vi "MoveXYZ.vi"(8 "error in (no error)":errorcluster, 9 "Destination coordinate":dbl[](array[numeric]), 10 "Notifiers":T1, 11 "Message Queues in":T14) -> (0 "error out":errorcluster)   [LabVIEW 2014]
uses:
  support/Message Queue/All Message Queues.ctl
  support/Message Queue/Message Cluster.ctl
  support/Notifiers/Notifiers.ctl
  support/Message Handler Loop Notifiers.ctl
  Parameter Analyzer/Parameter Analyzer Notifiers.ctl
  Switching Matrix/Switching Matrix Notifiers.ctl
  Stress Control/StressControl Notifiers.ctl
  Spectrometer/Spectrometer Notifiers.ctl
  Switches and Mirrors/SwitchesMirrors Notifiers.ctl
  Camera/Camera Notifiers.ctl
  XYZ Stage/XYZ Notifications.ctl
  Autofocus Notifiers.ctl
  Measurements/Optoelectronic Measurement/Optoelectronic Notifiers.ctl
  Measurements/Save Data/SaveData Notifiers.ctl
  Measurements/Instrument Sequence/Instrument Sequence Notifiers.ctl
  XYZ Stage/XYZ Config.ctl
  XYZ Stage/XYZ Connection Settings.ctl
  XYZ Stage/XYZ Stage Control.ctl
  XYZ Stage/XYZ Coordinate Control.ctl
  support/Message Queue/Message Queue.lvlib
panel:
  # "LICENSED MATERIALS – PROPERTY OF IBM\nCopyright IBM Corp. 2016, 2016\nALL RIGHTS RESERVED"
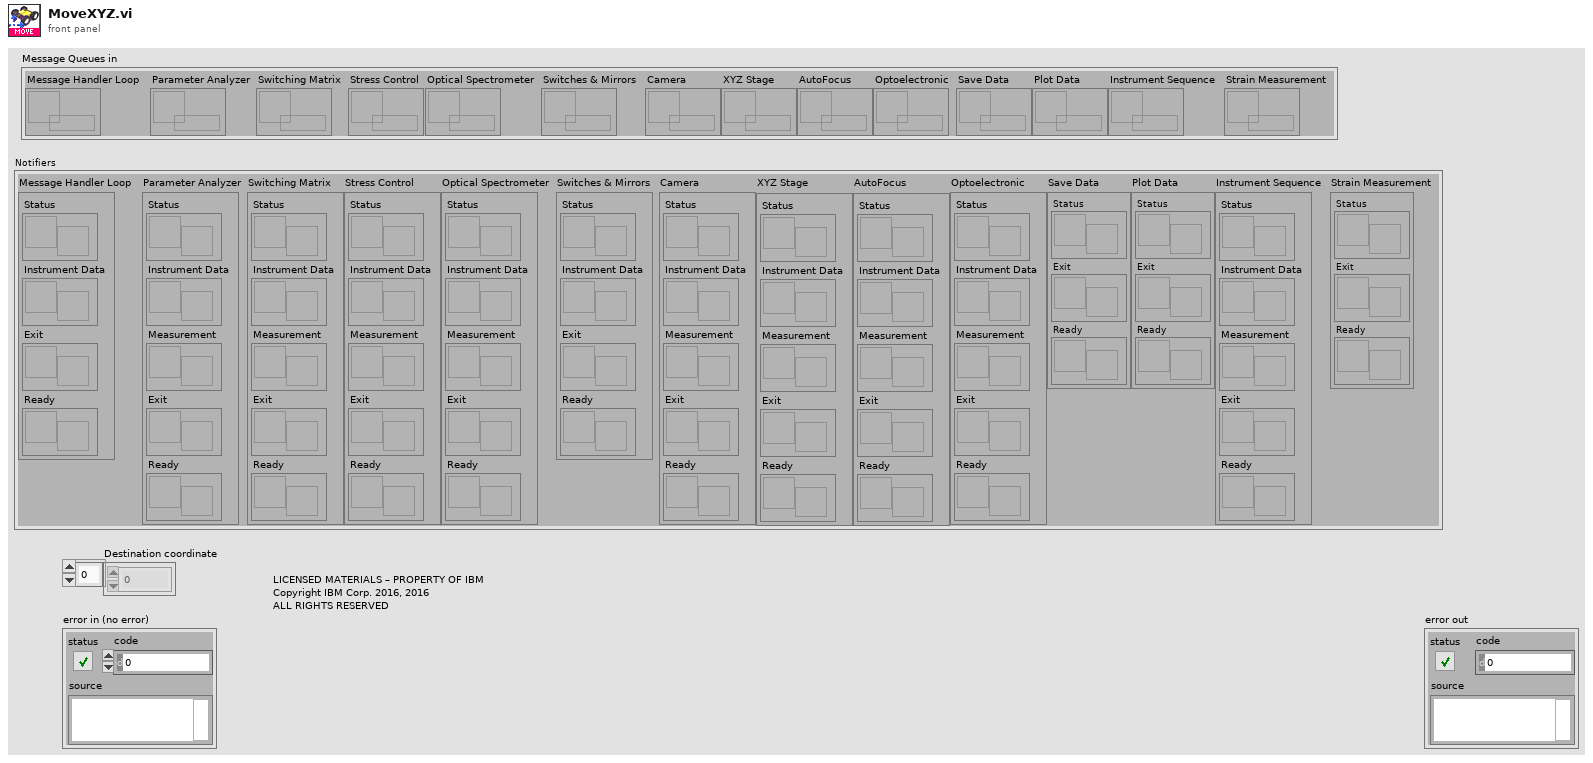
[diagram p1: front panel]
types:
  T1 = typedef "Notifiers.ctl" = cluster{"Message Handler Loop":T2, "Parameter Analyzer":T3, "Switching Matrix":T4, "Stress Control":T5, "Optical Spectrometer":T6, "Switches & Mirrors":T7, "Camera":T8, "XYZ Stage":T9, "AutoFocus":T10, "Optoelectronic":T11, "Save Data":T12, "Plot Data":T12, "Instrument Sequence":T13, "Strain Measurement":cluster{"Status":refnum<notifier>, "Exit":refnum<notifier>, "Ready":refnum<notifier>}}
  T2 = typedef "Message Handler Loop Notifiers.ctl" = cluster{"Status":refnum<notifier>, "Instrument Data":refnum<notifier>, "Exit":refnum<notifier>, "Ready":refnum<notifier>}
  T3 = typedef "Parameter Analyzer Notifiers.ctl" = cluster{"Status":refnum<notifier>, "Instrument Data":refnum<notifier>, "Measurement":refnum<notifier>, "Exit":refnum<notifier>, "Ready":refnum<notifier>}
  T4 = typedef "Switching Matrix Notifiers.ctl" = cluster{"Status":refnum<notifier>, "Instrument Data":refnum<notifier>, "Measurement":refnum<notifier>, "Exit":refnum<notifier>, "Ready":refnum<notifier>}
  T5 = typedef "StressControl Notifiers.ctl" = cluster{"Status":refnum<notifier>, "Instrument Data":refnum<notifier>, "Measurement":refnum<notifier>, "Exit":refnum<notifier>, "Ready":refnum<notifier>}
  T6 = typedef "Spectrometer Notifiers.ctl" = cluster{"Status":refnum<notifier>, "Instrument Data":refnum<notifier>, "Measurement":refnum<notifier>, "Exit":refnum<notifier>, "Ready":refnum<notifier>}
  T7 = typedef "SwitchesMirrors Notifiers.ctl" = cluster{"Status":refnum<notifier>, "Instrument Data":refnum<notifier>, "Exit":refnum<notifier>, "Ready":refnum<notifier>}
  T8 = typedef "Camera Notifiers.ctl" = cluster{"Status":refnum<notifier>, "Instrument Data":refnum<notifier>, "Measurement":refnum<notifier>, "Exit":refnum<notifier>, "Ready":refnum<notifier>}
  T9 = typedef "XYZ Notifications.ctl" = cluster{"Status":refnum<notifier>, "Instrument Data":refnum<notifier>, "Measurement":refnum<notifier>, "Exit":refnum<notifier>, "Ready":refnum<notifier>}
  T10 = typedef "Autofocus Notifiers.ctl" = cluster{"Status":refnum<notifier>, "Instrument Data":refnum<notifier>, "Measurement":refnum<notifier>, "Exit":refnum<notifier>, "Ready":refnum<notifier>}
  T11 = typedef "Optoelectronic Notifiers.ctl" = cluster{"Status":refnum<notifier>, "Instrument Data":refnum<notifier>, "Measurement":refnum<notifier>, "Exit":refnum<notifier>, "Ready":refnum<notifier>}
  T12 = typedef "SaveData Notifiers.ctl" = cluster{"Status":refnum<notifier>, "Exit":refnum<notifier>, "Ready":refnum<notifier>}
  T13 = typedef "Instrument Sequence Notifiers.ctl" = cluster{"Status":refnum<notifier>, "Instrument Data":refnum<notifier>, "Measurement":refnum<notifier>, "Exit":refnum<notifier>, "Ready":refnum<notifier>}
  T14 = typedef "Message Queue.lvlib/All Message Queues.ctl" = cluster{"Message Handler Loop":refnum<queue>, "Parameter Analyzer":refnum<queue>, "Switching Matrix":refnum<queue>, "Stress Control":refnum<queue>, "Optical Spectrometer":refnum<queue>, "Switches & Mirrors":refnum<queue>, "Camera":refnum<queue>, "XYZ Stage":refnum<queue>, "AutoFocus":refnum<queue>, "Optoelectronic":refnum<queue>, "Save Data":refnum<queue>, "Plot Data":refnum<queue>, "Instrument Sequence":refnum<queue>, "Strain Measurement":refnum<queue>}
  T15 = typedef "XYZ Config.ctl" = cluster{"Connection Settings":T16, "Manual Control":T17, "Coordinate Control":T18}
  T16 = typedef "XYZ Connection Settings.ctl" = cluster{"Tango VISA":refnum<visa-resource-name>, "Baudrate":i32, "Show Protocol?":bool}
  T17 = typedef "XYZ Stage Control.ctl" = cluster{"North":bool, "South":bool, "West":bool, "East":bool, "Up":bool, "Down":bool, "Stop":bool, "XY Step":dbl, "Z step":dbl}
  T18 = typedef "XYZ Coordinate Control.ctl" = cluster{"Motion Mode":enum16{"Absolute", "Relative"}, "Destination [mm]":dbl[]}
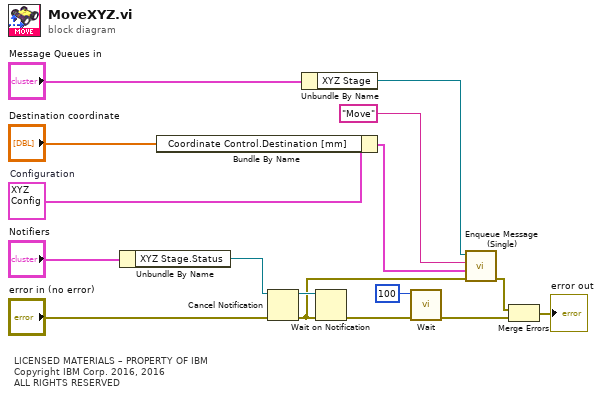
[diagram p0: block diagram]
diagram:
  w9 = T15 {"Connection Settings"={"Tango VISA"="", "Baudrate"=57600, "Show Protocol?"=FALSE}, "Manual Control"={"North"=FALSE, "South"=FALSE, "West"=FALSE, "East"=FALSE, "Up"=FALSE, "Down"=FALSE, "Stop"=FALSE, "XY Step"=0.0, "Z step"=0.0}, "Coordinate Control"={"Motion Mode"=enum."Absolute", "Destination [mm]"=[]}}  # Configuration
  # "LICENSED MATERIALS – PROPERTY OF IBM\nCopyright IBM Corp. 2016, 2016\nALL RIGHTS RESERVED"
  n1 = Unbundle By Name("Notifiers") -> ("XYZ Stage.Status"=w3:refnum<notifier>)
  n2 = Bundle By Name(cluster=w9, "Coordinate Control.Destination [mm]"="Destination coordinate") -> (w10:T15)
  n3 = Cancel Notification(0:w3, 3:"error in (no error)") -> (8:w5:refnum<notifier>, 11:w4:errorcluster)  [unwired: 1 out]
  n4 = Unbundle By Name("Message Queues in") -> ("XYZ Stage"=w11:refnum<queue>)
  n5 = Wait on Notification(notifier=w5, error in (no error)=w4) -> (error out=w7:errorcluster)  [unwired: 2 in, 3 out]
  n6 = call "Wait.vi"("error in (no error)"=w7, "milliseconds to wait"=u32 100) -> ("error out"=w8:errorcluster)  [unwired: 9 in]
  n7 = call "Enqueue Message (Single).vi"("error in (no error)"=w4, "Message Data"=w10, "Message"="Move", "Message Queue"=w11) -> ("error out"=w1:errorcluster)  [unwired: 7 out]
  n8 = Merge Errors(w1, w8) -> (→"error out":errorcluster)
